vi "SRV_About - LPD Application.vi"(9 "Close Timeout ms (none)":i32=-1, 10 "Version Info":string, 11 "Application Name":string="LPD Application") -> ()   [LabVIEW 2014]
doc: "This VI is used to display information about the system.\n\nNote: The close button is transparent. To edit the System/Project name and other info, move the Close button to \"back\" and make your changes. After making changes, move the Close button to \"front.\"\n\n<B>Inputs:</B>\nApplication Name: This string is used to identify the name of the app.\n\nVersion Info: This string input is used to accept version information that is displayed in the about window.\n\nClose Timeout ms(none): This I32 is used to define how long the about window is displayed. If unwired , the value is -1 (no timeout) and the window will stay open until the user clicks in the window.\n\n\nAuthor: Mike Schultz (mschultz11711@gmail.com)"
panel:
  in  "Close":bool
  out "Version":string
  # "Click in window to close."
  # "This application was developed by Mike Schultz (mschultz11711@gmail.com)"
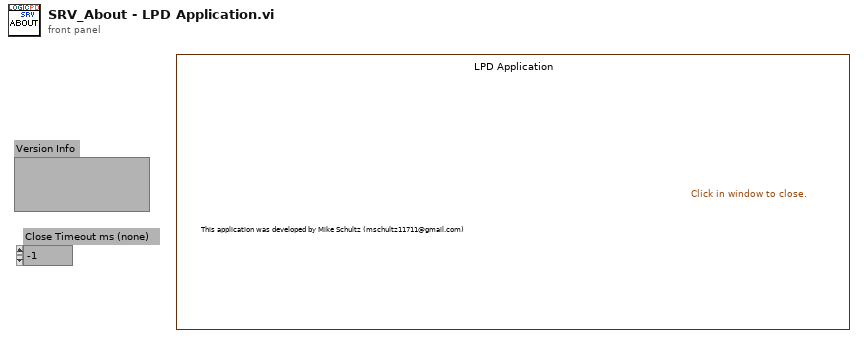
[diagram p1: front panel]
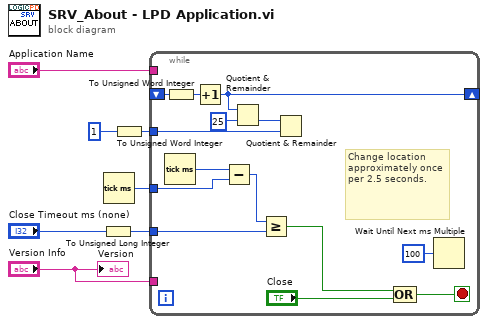
[diagram p0: block diagram]
diagram:
  n1 = To Unsigned Long Integer(number="Close Timeout ms (none)") -> (unsigned 32bit integer=w4:u32)
  n2 = Tick Count (ms)() -> (millisecond timer value=w6:u32)
  n3 = To Unsigned Word Integer(number=u16 1) -> (unsigned 16bit integer=w2:u16)
  n4 = while {
    tunnel: "Application Name" -> [_]
    shift-left: _ -> [w14]
    shift-right: [w10] -> _
    tunnel: w4 -> [w15]
    tunnel: w6 -> [w19]
    tunnel: "Version Info" -> [_]
    tunnel: w2 -> [w8]
    stop <- w18 stop-if-true
    # "Change location approximately once per 2.5 seconds."
    n5 = Tick Count (ms)() -> (millisecond timer value=w20:u32)
    n6 = To Unsigned Word Integer(number=w14) -> (unsigned 16bit integer=w11:u16)
    n7 = Increment(x=w11) -> (x+1=w10:u16)
    n8 = Subtract(x=w20, y=w19) -> (x-y=w17:u32)
    n9 = Quotient & Remainder(x=w10, y=u16 25) -> (floor(x/y)=w12:u16)  [unwired: 1 out]
    n10 = Greater Or Equal?(x=w17, y=w15) -> (x >= y?=w16:bool)
    n11 = Quotient & Remainder(x=w12, y=w8) -> ()  [unwired: 2 out]
    n12 = Compound Arithmetic op=OR(w16, "Close") -> (w18:bool)
    n13 = Wait Until Next ms Multiple(millisecond multiple=u32 100) -> ()  [unwired: 1 out]
  }
  "Version" <- "Version Info"
